vi "GlobalGetHeidenhainDriftOnOff.vi"() -> ()   [LabVIEW 2011]
panel:
  out "GetDrift":bool
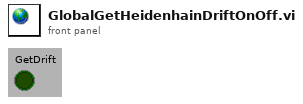
[diagram p1: front panel]
diagram:
